vi "Router - PXImc Intial Handshaking.vi"(5 "Reader Buffer Size In":u64, 6 "# Elements to Read":i32, 7 "Connection Timeout (s)":dbl, 8 "error in (no error)":errorcluster, 9 "Reader Conn ID":u16, 10 "Writer Conn ID":u16, 11 "Resource Name In":string) -> (0 "error out":errorcluster, 2 "Data Out":u32[](array[numeric]))   [LabVIEW 2016, in "PXImc Router.lvlib"]
uses:
  PXImc Router.lvlib
  <vilib>/pximc/Initialize Reader Session (U32).vi
  <vilib>/pximc/Initialize Writer Session (U32).vi
  <vilib>/pximc/Connect (U32).vi
  <vilib>/pximc/Read (U32).vi
  <vilib>/pximc/Write (U32).vi
  <vilib>/pximc/nipximc.lvlib
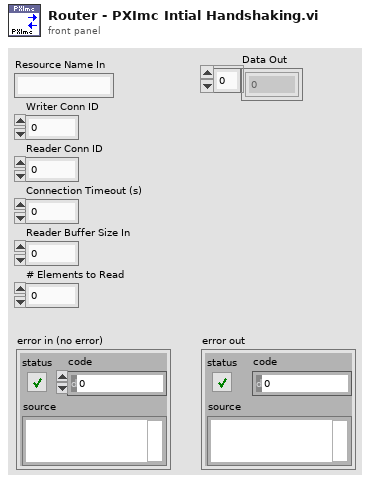
[diagram p1: front panel]
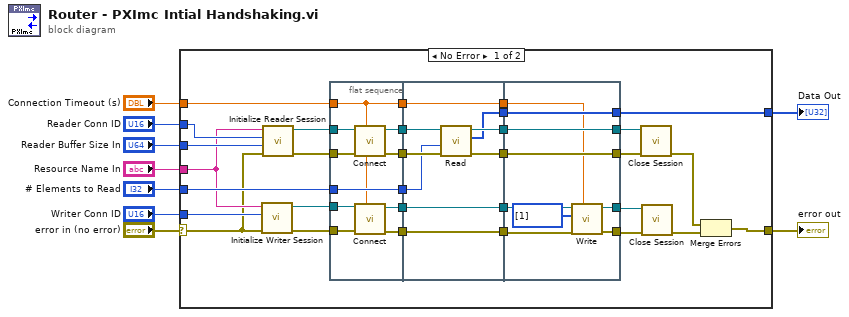
[diagram p0: block diagram]
diagram:
  n1 = case shown="No Error" "error in (no error)" {
    selector: "error in (no error)" -> [w12 w69]
    tunnel: "# Elements to Read" -> [w30 _]
    tunnel: "Reader Conn ID" -> [w29 _]
    tunnel: "Writer Conn ID" -> [w28 _]
    tunnel: "Reader Buffer Size In" -> [w27 _]
    tunnel: "Resource Name In" -> [w26 _]
    tunnel: [w25 _] -> w4
    tunnel: "Connection Timeout (s)" -> [w24 _]
    tunnel: [w19 w69] -> w2
    frame No Error {
      n2 = call-poly <vilib>:"Initialize Writer Session.vi"("error in (no error)"=w12, "connection id (1)"=w28, "interface"=w26) -> ("error out"=w16:errorcluster, "session out"=w15:refnum<k21>)  [unwired: 7 in]
      n3 = call-poly <vilib>:"Initialize Reader Session.vi"("error in (no error)"=w12, "buffer size"=w27, "writer's connection id (1)"=w29, "interface"=w26) -> ("error out"=w14:errorcluster, "session out"=w13:refnum<k21>)  [unwired: 6 in]
      n4 = flat-sequence {
        tunnel: w13 -> [w50]
        tunnel: w14 -> [w49]
        tunnel: w15 -> [w46]
        tunnel: w16 -> [w45]
        tunnel: [w48] -> w40
        tunnel: [w47] -> w39
        tunnel: [w44] -> w38
        tunnel: [w43] -> w37
        tunnel: w24 -> [w41]
        tunnel: w30 -> [w42]
        tunnel: [w42] -> w36
        tunnel: [w41] -> w11
        tunnel: w40 -> [w57]
        tunnel: w39 -> [w55]
        tunnel: w38 -> [w59]
        tunnel: w37 -> [w58]
        tunnel: [w56] -> w35
        tunnel: [w54] -> w34
        tunnel: [w59] -> w33
        tunnel: [w58] -> w32
        tunnel: [w53] -> w31
        tunnel: w36 -> [w52]
        tunnel: w11 -> [w51]
        tunnel: [w51] -> w10
        tunnel: [w67] -> w23
        tunnel: [w68] -> w22
        tunnel: w35 -> [w68]
        tunnel: w34 -> [w67]
        tunnel: w33 -> [w65]
        tunnel: w32 -> [w66]
        tunnel: [w64] -> w21
        tunnel: [w63] -> w20
        tunnel: w31 -> [w61]
        tunnel: [w61] -> w25
        tunnel: w10 -> [w60]
        frame #0 {
          n5 = call-poly <vilib>:"Connect.vi"("timeout in seconds (-1)"=w41, "error in (no error)"=w49, "session in"=w50) -> ("error out"=w47:errorcluster, "session out"=w48:refnum<k21>)  [unwired: 7 in]
          n6 = call-poly <vilib>:"Connect.vi"("timeout in seconds (-1)"=w41, "error in (no error)"=w45, "session in"=w46) -> ("error out"=w44:errorcluster, "session out"=w43:refnum<k21>)  [unwired: 7 in]
        }
        frame #1 {
          n7 = call-poly <vilib>:"Read.vi"("error in (no error)"=w55, "number of elements"=w52, "session in"=w57) -> ("error out"=w54:errorcluster, "data"=w53:u32[], "session out"=w56:refnum<k21>)  [unwired: 6 in]
        }
        frame #2 {
          n8 = call-poly <vilib>:"Write.vi"("timeout in seconds (5)"=w60, "error in (no error)"=w65, "data"=u32[] [1], "session in"=w66) -> ("error out"=w64:errorcluster, "session out"=w63:refnum<k21>)  [unwired: 5 in, 1 out]
        }
      }
      n9 = call <vilib>:"Close Session.vi"("error in (no error)"=w23, "session in"=w22) -> ("error out"=w17:errorcluster)  [unwired: 9 in]
      n10 = call <vilib>:"Close Session.vi"("error in (no error)"=w21, "session in"=w20) -> ("error out"=w18:errorcluster)  [unwired: 9 in]
      n11 = Merge Errors(w17, w18) -> (w19:errorcluster)
    }
    frame Error {
    }
  }
  "Data Out" <- w4
  "error out" <- w2
